vi "Read all OSA params.vi"(8 "error in (no error)":errorcluster, 11 "VISA resource name":refnum<visa-resource-name>) -> (0 "error out":errorcluster, 2 "total read":string[](array[string]), 3 "VISA resource name out":refnum<visa-resource-name>)   [LabVIEW 2021, in "Ceyear.lvlib"]
doc: "Reads a trace from the spectrum analyzer."
uses:
  <instrlib>/Ceyear/Ceyear.lvlib
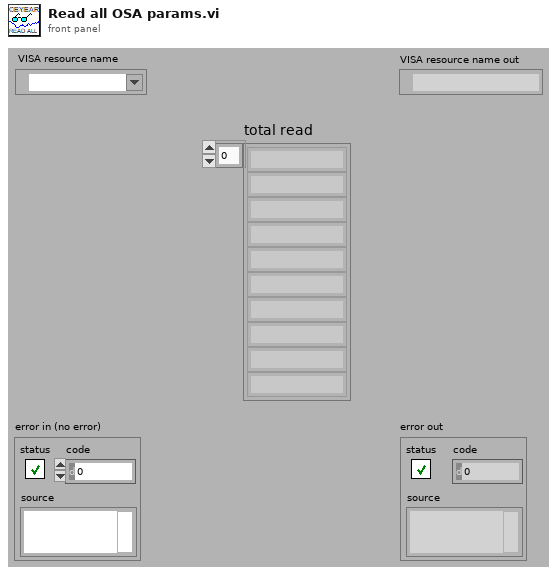
[diagram p1: front panel]
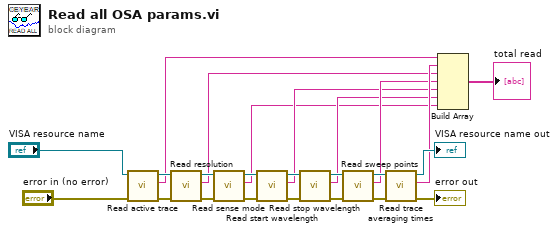
[diagram p0: block diagram]
diagram:
  n1 = call <instrlib>:"Read active trace.vi"("error in (no error)"="error in (no error)", "VISA resource name"="VISA resource name") -> ("error out"=w21:errorcluster, "Active trace"=w8:string, "VISA resource name out"=w22:refnum<visa-resource-name>)  [unwired: 7 in]
  n2 = call <instrlib>:"Read resolution.vi"("error in (no error)"=w21, "VISA resource name"=w22) -> ("error out"=w19:errorcluster, "Resolution"=w6:string, "VISA resource name out"=w20:refnum<visa-resource-name>)  [unwired: 7 in]
  n3 = call <instrlib>:"Read sense mode.vi"("error in (no error)"=w19, "VISA resource name"=w20) -> ("error out"=w17:errorcluster, "Mode"=w2:string, "VISA resource name out"=w18:refnum<visa-resource-name>)  [unwired: 7 in]
  n4 = call <instrlib>:"Read start wavelength.vi"("error in (no error)"=w17, "VISA resource name"=w18) -> ("error out"=w15:errorcluster, "Start wavelength"=w4:string, "VISA resource name out"=w16:refnum<visa-resource-name>)  [unwired: 7 in]
  n5 = call <instrlib>:"Read stop wavelength.vi"("error in (no error)"=w15, "VISA resource name"=w16) -> ("error out"=w13:errorcluster, "Stop wavelength"=w3:string, "VISA resource name out"=w14:refnum<visa-resource-name>)  [unwired: 7 in]
  n6 = call <instrlib>:"Read sweep points.vi"("error in (no error)"=w13, "VISA resource name"=w14) -> ("error out"=w11:errorcluster, "Points"=w5:string, "VISA resource name out"=w12:refnum<visa-resource-name>)  [unwired: 7 in]
  n7 = call <instrlib>:"Read trace averaging times.vi"("error in (no error)"=w11, "VISA resource name"=w12) -> ("error out"=→"error out":errorcluster, "Averaging times"=w7:string, "VISA resource name out"=→"VISA resource name out":refnum<visa-resource-name>)  [unwired: 7 in]
  n8 = Build Array(w8, w7, w6, w5, w4, w3, w2) -> (→"total read":string[])
